vi "Serial Ploter.vi"() -> ()   [LabVIEW 2018]
uses:
  <vilib>/Instr/_visa.llb/VISA Configure Serial Port (Instr).vi
  <vilib>/Utility/file.llb/Write Delimited Spreadsheet (string).vi
  <vilib>/Utility/file.llb/Write Delimited Spreadsheet (DBL).vi
panel:
  out "transposed array":dbl[][](array[numeric])
  out "Time":dbl
  in  "String":string="D:\\Dizertatie\\Analiza-inteligenta-a-mersului-main\\Analiza-inteligenta-a-mersului-main\\data\\"
  in  "Activitatea":ext
  in  "Numarul persoanei":ext
  in  "Timer[s]":dbl
  out "GyroY":dbl(graph)
  out "GyroX":dbl(graph)
  out "X":dbl(graph)
  out "Y":dbl(graph)
  out "read buffer":string
  in  "stop":bool
  in  "VISA resource name":refnum<visa-resource-name>
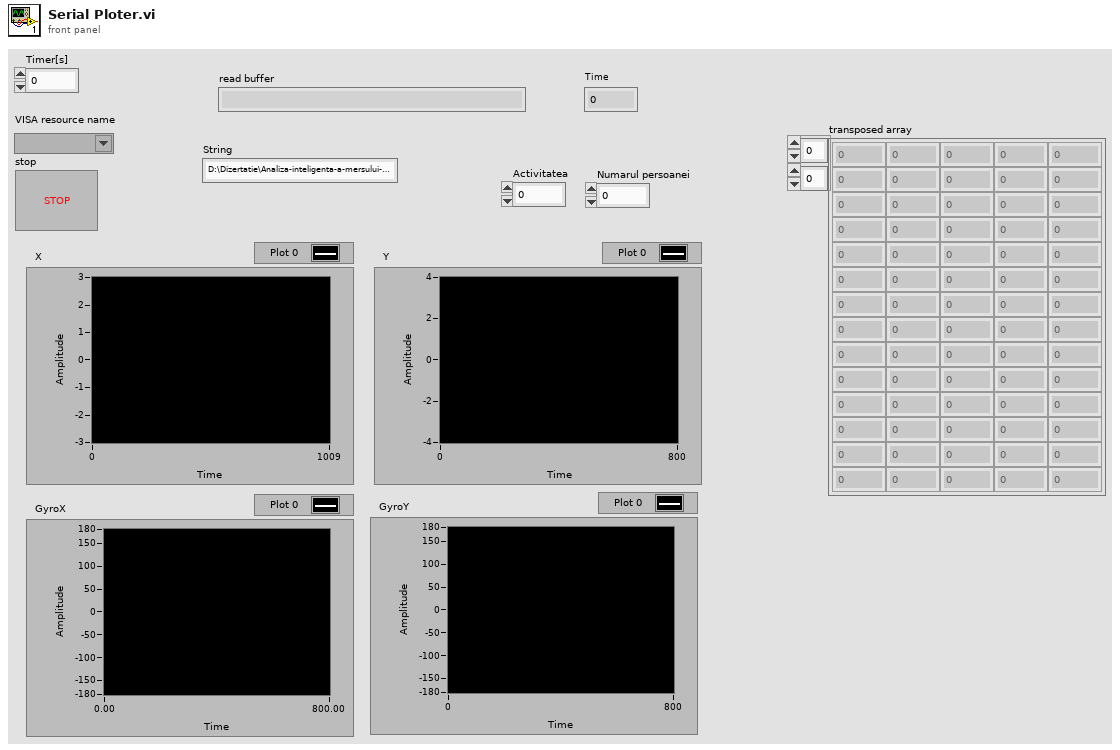
[diagram p1: front panel]
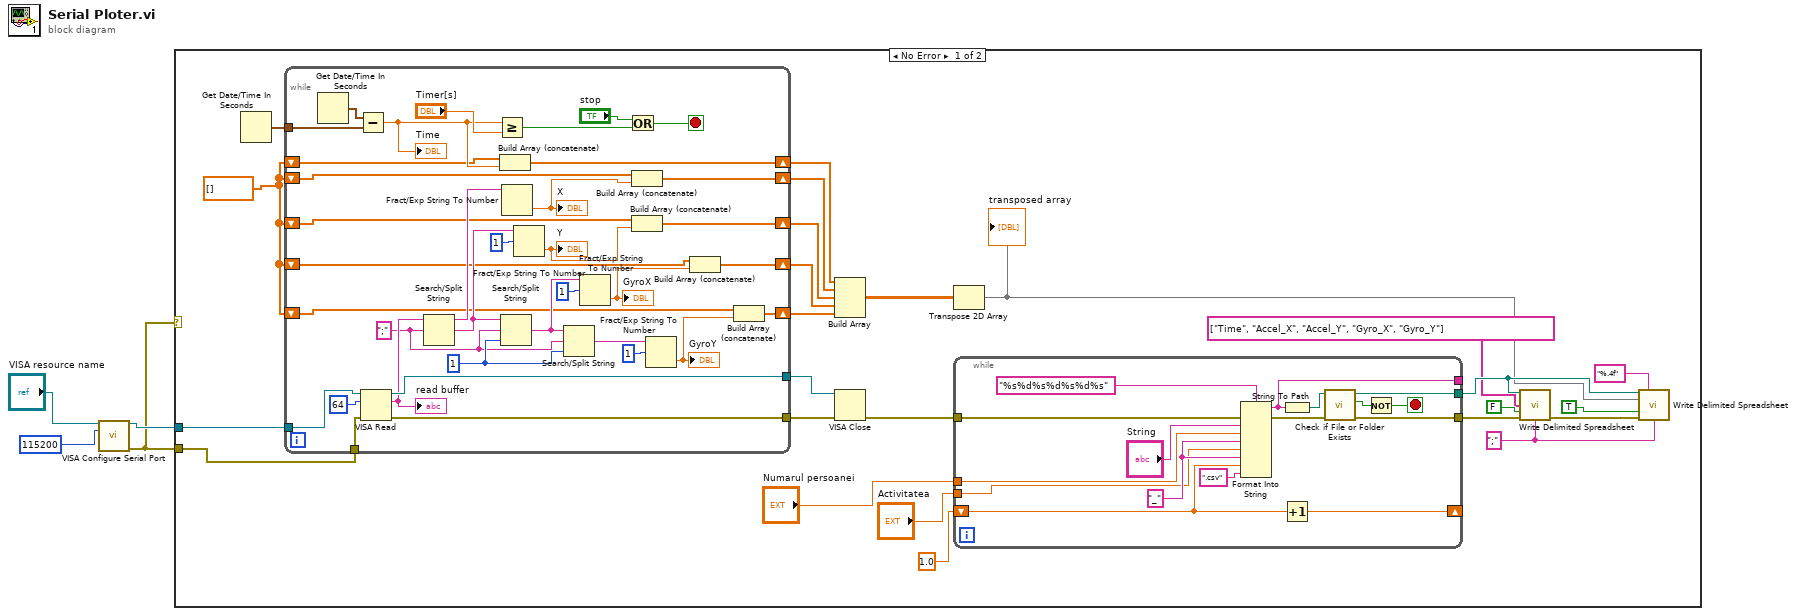
[diagram p0: block diagram]
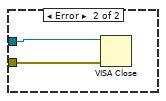
[diagram p2: hidden frame]
diagram:
  n1 = call-poly "VISA Configure Serial Port"("VISA resource name"="VISA resource name", "baud rate (9600)"=u32 115200) -> ("VISA resource name out"=w2:refnum<visa-resource-name>, "error out"=w1:errorcluster)  [unwired: 12 in]
  n2 = case shown="No Error" w1 {
    tunnel: w2 -> [w6 w83]
    tunnel: w1 -> [w5 w82]
    frame No Error {
      w7 = dbl[] []
      w19 = ";" ("delimiter (\\t)")
      n3 = Get Date/Time In Seconds() -> (seconds since 1Jan1904=w27:timestamp)
      n4 = while {
        tunnel: [w80] -> w29
        tunnel: [w79] -> w28
        tunnel: w27 -> [w68]
        shift-right: [w62] -> w26
        shift-left: w7 -> [w61]
        shift-right: [w59] -> w25
        shift-left: w7 -> [w58]
        shift-right: [w56] -> w24
        shift-left: w7 -> [w55]
        shift-right: [w53] -> w23
        shift-left: w7 -> [w52]
        shift-right: [w49] -> w8
        shift-left: w7 -> [w48]
        tunnel: w6 -> [w47]
        tunnel: w5 -> [w46]
        stop <- w51 stop-if-true
        w74 = 1 ("offset (0)")
        w73 = ";" ("search string/char (-)")
        n5 = Get Date/Time In Seconds() -> (seconds since 1Jan1904=w67:timestamp)
        n6 = Subtract(x=w67, y=w68) -> (x-y=w50:dbl)
        "Time" <- w50
        n7 = VISA Read(VISA resource name=w47, byte count=u32 64, error in (no error)=w46) -> (VISA resource name out=w79:refnum<visa-resource-name>, read buffer=w78:string, error out=w80:errorcluster)  [unwired: 1 out]
        "read buffer" <- w78
        n8 = Search/Split String(string=w78, search string/char (-)=w73) -> (substring before match=w76:string, match + rest of string=w75:string)  [unwired: 1 in, 1 out]
        n9 = Greater Or Equal?(x=w50, y="Timer[s]") -> (x >= y?=w64:bool)
        n10 = Build Array (concatenate)(w48, w50) -> (w49:dbl[])
        n11 = Search/Split String(string=w75, search string/char (-)=w73, offset (0)=w74) -> (match + rest of string=w72:string)  [unwired: 2 out]
        n12 = Fract/Exp String To Number(string=w76) -> (number=w63:dbl)  [unwired: 3 in, 1 out]
        "X" <- w63
        n13 = Fract/Exp String To Number(string=w75, offset=1) -> (number=w60:dbl)  [unwired: 2 in, 1 out]
        "Y" <- w60
        n14 = Search/Split String(string=w72, search string/char (-)=w73, offset (0)=w74) -> (match + rest of string=w70:string)  [unwired: 2 out]
        n15 = Fract/Exp String To Number(string=w72, offset=1) -> (number=w57:dbl)  [unwired: 2 in, 1 out]
        "GyroX" <- w57
        n16 = Or(x="stop", y=w64) -> (x .or. y?=w51:bool)
        n17 = Build Array (concatenate)(w61, w63) -> (w62:dbl[])
        n18 = Build Array (concatenate)(w58, w60) -> (w59:dbl[])
        n19 = Fract/Exp String To Number(string=w70, offset=1) -> (number=w54:dbl)  [unwired: 2 in, 1 out]
        "GyroY" <- w54
        n20 = Build Array (concatenate)(w55, w57) -> (w56:dbl[])
        n21 = Build Array (concatenate)(w52, w54) -> (w53:dbl[])
      }
      n22 = Build Array(w8, w26, w25, w24, w23) -> (w22:dbl[][])
      n23 = VISA Close(VISA resource name=w28, error in (no error)=w29) -> (error out=w13:errorcluster)
      n24 = Transpose 2D Array(2D array=w22) -> (transposed array=w10:dbl[][])
      "transposed array" <- w10
      n25 = while {
        tunnel: "Numarul persoanei" -> [w44]
        tunnel: "Activitatea" -> [w41]
        shift-right: [w35] -> _
        shift-left: 1.0 -> [w36]
        tunnel: [w34] -> w15
        tunnel: w13 -> [w33]
        tunnel: [w32] -> w17
        tunnel: [w30] -> _
        stop <- w38 stop-if-true
        w42 = "_"
        n26 = Format Into String(format string="%s%d%s%d%s%d%s", error in=w33, "String", w44, w42, w41, w42, w36, ".csv" ("input 7")) -> (resulting string=w30:string, error out=w37:errorcluster)  [unwired: 1 in]
        n27 = String To Path(string=w30) -> (path=w40:path)
        n28 = Increment(x=w36) -> (x+1=w35:dbl)
        n29 = call <vilib>:"Check if File or Folder Exists.vi"("error in (no error)"=w37, "path"=w40) -> ("error out"=w34:errorcluster, "file or folder exists?"=w39:bool, "dup path"=w32:path)  [unwired: 7 in]
        n30 = Not(x=w39) -> (.not. x?=w38:bool)
      }
      n31 = call-poly <vilib>:"Write Delimited Spreadsheet.vi"("file path (dialog if empty)"=w17, "1D data"=string[] ["Time", "Accel_X", "Accel_Y", "Gyro_X", "Gyro_Y"] ("Array"), "append to file? (new file:F)"=FALSE, "error in (no error)"=w15, "delimiter (\\t)"=w19) -> ("error out"=w16:errorcluster)  [unwired: 9 in, 1 out]
      n32 = call-poly <vilib>:"Write Delimited Spreadsheet.vi"("file path (dialog if empty)"=w17, "format (%.3f)"="%.4f", "2D data"=w10, "append to file? (new file:F)"=TRUE, "error in (no error)"=w16, "delimiter (\\t)"=w19) -> ()  [unwired: 8 in, 2 out]
    }
    frame Error {
      n33 = VISA Close(VISA resource name=w83, error in (no error)=w82) -> ()  [unwired: 1 out]
    }
  }
